vi "OpenAndRunVi (SubVI).vi"(11 "VI in":refnum<vi>) -> ()   [LabVIEW 2017]
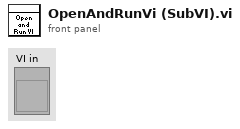
[diagram p1: front panel]
types:
  T1 = enum32{"Invalid", "Standard", "Closed", "Hidden", "Minimized", "Maximized"}
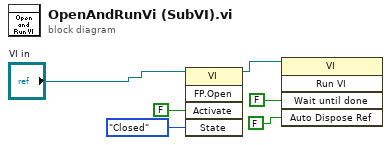
[diagram p0: block diagram]
diagram:
  n1 = invoke class="VI" method="FP.Open"(reference="VI in", "Activate"=FALSE ("Activate?"), "State"=T1."Closed") -> (reference out=w5:refnum<vi>)  [unwired: 2 in, 4 out]
  n2 = invoke class="VI" method="Run VI"(reference=w5, "Wait until done"=FALSE ("Wait Until Done"), "Auto Dispose Ref"=FALSE ("Wait Until Done")) -> ()  [unwired: 2 in, 5 out]
